vi "Close.vi"(8 "error in (no error)":errorcluster, 11 "Endpoint in":refnum<class "Endpoint.lvclass">) -> (0 "error out":errorcluster, 3 "Endpoint out":refnum<class "Endpoint.lvclass">)   [LabVIEW 2020, in "Stream.lvlib" / "Endpoint.lvclass"]
uses:
  Endpoint.lvclass
  Endpoint.lvclass/Endpoint.ctl
  <vilib>/Utility/error.llb/Error Cluster From Error Code.vi
  <vilib>/ErrorRing/Error Ring.xnode
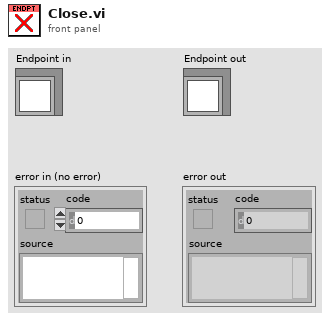
[diagram p1: front panel]
types:
  T1 = typedef "Stream.lvlib/Endpoint.lvclass/Ref Data.ctl" = cluster{"URI":refnum<class "URI.lvclass">, "State Callbacks":T2[], "Open":bool, "Sniffer Callbacks":T2[]}
  T2 = typedef "Stream.lvlib/Endpoint.lvclass/State Callback.ctl" = cluster{"Owner":refnum<class>, "VI":refnum<vi>}
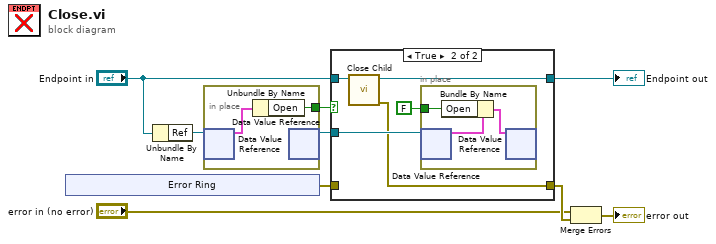
[diagram p0: block diagram]
diagram:
  n1 = xnode "Error Ring"() -> ("error out"=w6:errorcluster)
  n2 = Unbundle By Name("Endpoint in") -> ("Ref"=w9:refnum<data-value>)
  n3 = in-place {
    in-place-border: [w10] -> w8
    n4 = in-place-dvr #1(w9) -> (w11:T1)  [unwired: 1 out]
    n5 = Unbundle By Name(w11) -> ("Open"=w10:bool)
    n6 = in-place-dvr #1() -> (w7:refnum<data-value>)  [unwired: 1 in, 1 out]
  }
  n7 = case shown="True" w8 {
    tunnel: "Endpoint in" -> [w13 w18]
    tunnel: w7 -> [_ w16]
    tunnel: [w13 w17] -> w4
    tunnel: [w12 w15] -> w5
    tunnel: w6 -> [w12 _]
    frame False {
    }
    frame True {
      n8 = call-dynamic "Close Child.vi"("Endpoint in"=w18) -> ("error out"=w15:errorcluster, "Endpoint out"=w17:refnum<class "Endpoint.lvclass">)  [unwired: 9 in]
      n9 = in-place {
        in-place-border: FALSE ("status") -> [w19]
        n10 = in-place-dvr #2(w16) -> (w21:T1)  [unwired: 1 out]
        n11 = Bundle By Name(cluster=w21, "Open"=w19) -> (w20:T1)
        n12 = in-place-dvr #2(w20) -> ()  [unwired: 2 out]
      }
    }
  }
  "Endpoint out" <- w4
  n13 = Merge Errors("error in (no error)", w5) -> (→"error out":errorcluster)
